vi "PlotStateMachine.vi"   [LabVIEW 2020]
types:
  T1 = enum16{"_Quit_", "Init", "load", "Pin-Mix", "Trace-Show/Hide", "Unit-Change", "Display/Print", "Exit"}
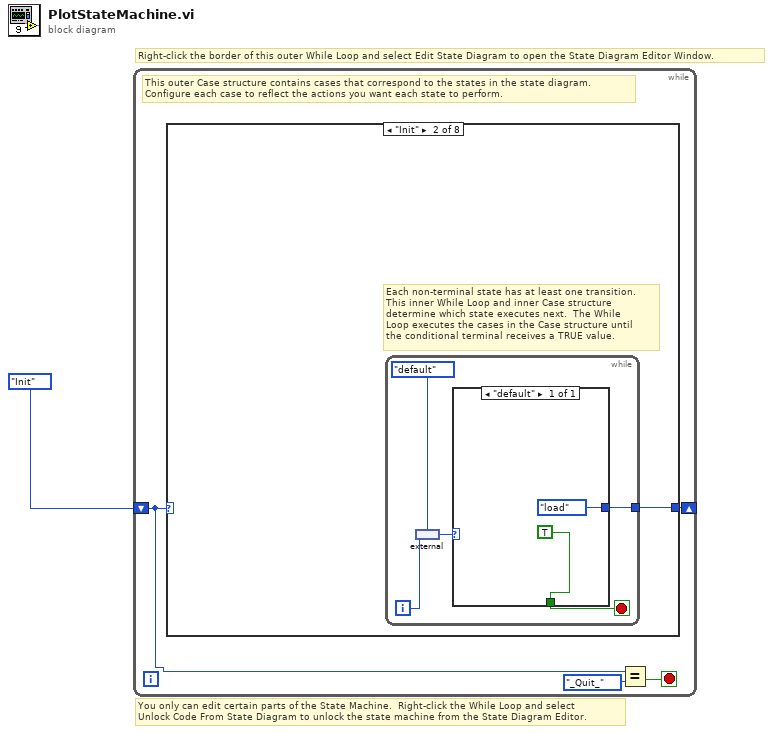
[diagram p0: block diagram]
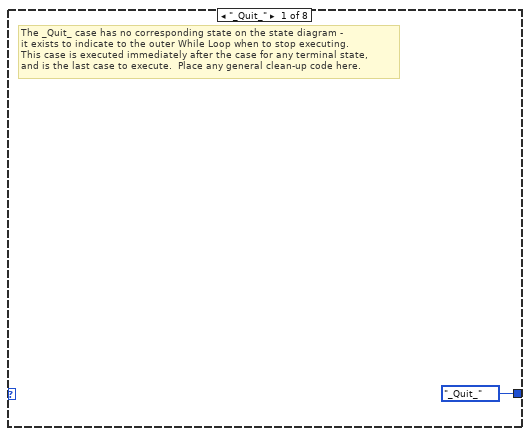
[diagram p2: hidden frame]
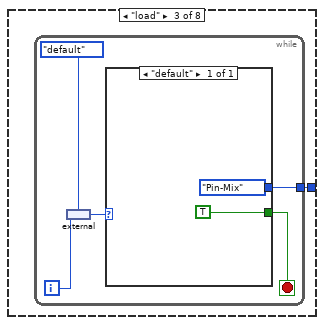
[diagram p3: hidden frame]
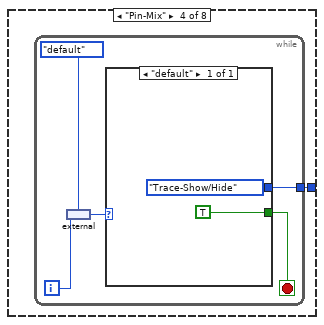
[diagram p4: hidden frame]
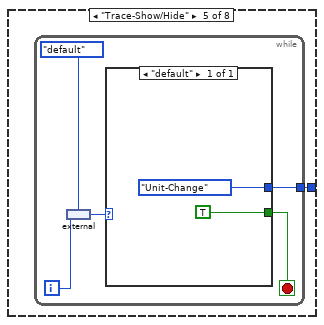
[diagram p5: hidden frame]
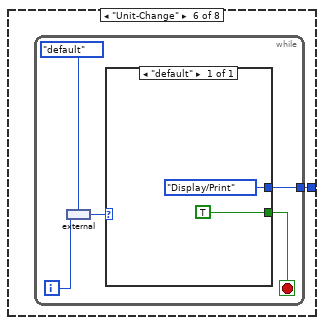
[diagram p6: hidden frame]
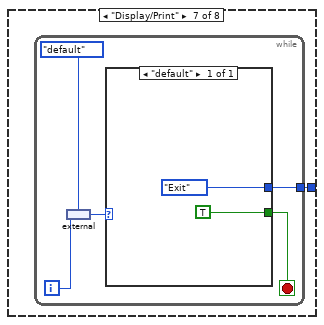
[diagram p7: hidden frame]
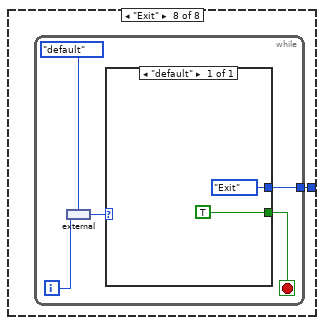
[diagram p8: hidden frame]
diagram:
  # "Right-click the border of this outer While Loop and select Edit State Diagram to open the State Diagram Editor Window."
  # "You only can edit certain parts of the State Machine.  Right-click the While Loop and select \nUnlock Code From State Diagram to unlock the state machine from the State Diagram Editor."
  n1 = while {
    shift-right: [w4] -> _
    shift-left: T1."Init" -> [w5]
    stop <- w3 stop-if-true
    # "This outer Case structure contains cases that correspond to the states in the state diagram.  \nConfigure each case to reflect the actions you want each state to perform."
    n2 = case shown="\"Init\"" w5 {
      tunnel: [T1."_Quit_" w7 w20 w33 w46 w59 w72 w85] -> w4
      frame "_Quit_" {
        # "The _Quit_ case has no corresponding state on the state diagram -\nit exists to indicate to the outer While Loop when to stop executing.\nThis case is executed immediately after the case for any terminal state, \nand is the last case to execute.  Place any general clean-up code here."
      }
      frame "Init" {
        # "Each non-terminal state has at least one transition.\nThis inner While Loop and inner Case structure \ndetermine which state executes next.  The While \nLoop executes the cases in the Case structure until \nthe conditional terminal receives a TRUE value."
        n3 = while {
          tunnel: [w9] -> w7
          i -> [w12]
          stop <- w8 stop-if-true
          n4 = external(enum16{"default"}."default", w12) -> (w10:enum16{"default"})
          n5 = case shown="\"default\"" w10 {
            tunnel: [T1."load"] -> w9
            tunnel: [TRUE] -> w8
            frame "default" {
            }
          }
        }
      }
      frame "load" {
        n6 = while {
          tunnel: [w22] -> w20
          i -> [w25]
          stop <- w21 stop-if-true
          n7 = external(enum16{"default"}."default", w25) -> (w23:enum16{"default"})
          n8 = case shown="\"default\"" w23 {
            tunnel: [T1."Pin-Mix"] -> w22
            tunnel: [TRUE] -> w21
            frame "default" {
            }
          }
        }
      }
      frame "Pin-Mix" {
        n9 = while {
          tunnel: [w35] -> w33
          i -> [w38]
          stop <- w34 stop-if-true
          n10 = external(enum16{"default"}."default", w38) -> (w36:enum16{"default"})
          n11 = case shown="\"default\"" w36 {
            tunnel: [T1."Trace-Show/Hide"] -> w35
            tunnel: [TRUE] -> w34
            frame "default" {
            }
          }
        }
      }
      frame "Trace-Show/Hide" {
        n12 = while {
          tunnel: [w48] -> w46
          i -> [w51]
          stop <- w47 stop-if-true
          n13 = external(enum16{"default"}."default", w51) -> (w49:enum16{"default"})
          n14 = case shown="\"default\"" w49 {
            tunnel: [T1."Unit-Change"] -> w48
            tunnel: [TRUE] -> w47
            frame "default" {
            }
          }
        }
      }
      frame "Unit-Change" {
        n15 = while {
          tunnel: [w61] -> w59
          i -> [w64]
          stop <- w60 stop-if-true
          n16 = external(enum16{"default"}."default", w64) -> (w62:enum16{"default"})
          n17 = case shown="\"default\"" w62 {
            tunnel: [T1."Display/Print"] -> w61
            tunnel: [TRUE] -> w60
            frame "default" {
            }
          }
        }
      }
      frame "Display/Print" {
        n18 = while {
          tunnel: [w74] -> w72
          i -> [w77]
          stop <- w73 stop-if-true
          n19 = external(enum16{"default"}."default", w77) -> (w75:enum16{"default"})
          n20 = case shown="\"default\"" w75 {
            tunnel: [T1."Exit"] -> w74
            tunnel: [TRUE] -> w73
            frame "default" {
            }
          }
        }
      }
      frame "Exit" {
        n21 = while {
          tunnel: [w87] -> w85
          i -> [w90]
          stop <- w86 stop-if-true
          n22 = external(enum16{"default"}."default", w90) -> (w88:enum16{"default"})
          n23 = case shown="\"default\"" w88 {
            tunnel: [T1."Exit"] -> w87
            tunnel: [TRUE] -> w86
            frame "default" {
            }
          }
        }
      }
    }
    n24 = Equal?(x=w5, y=T1."_Quit_") -> (x = y?=w3:bool)
  }
